vi "Limit Record Length.vi"(0 "Scope Reference":refnum<k15>, 11 "error in (no error)":errorcluster) -> (4 "Scope Reference Out":refnum<k15>, 15 "error out":errorcluster)   [LabVIEW 2020, in "LDO PSRR.lvlib"]
uses:
  LDO PSRR.lvlib
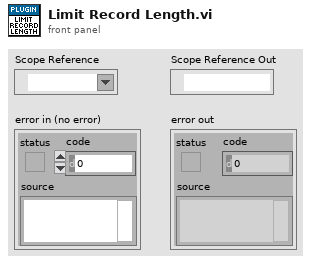
[diagram p1: front panel]
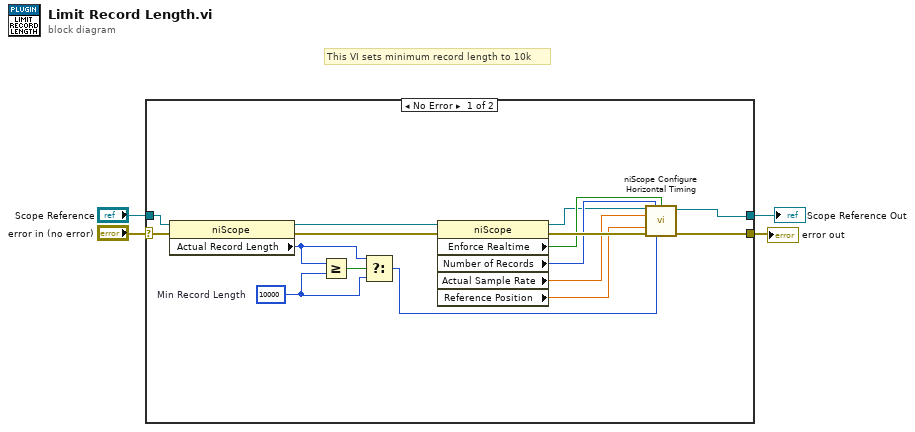
[diagram p0: block diagram]
diagram:
  # "This VI sets minimum record length to 10k"
  n1 = case shown="No Error" "error in (no error)" {
    selector: "error in (no error)" -> [w20 w22]
    tunnel: [w8 w22] -> w4
    tunnel: [w10 w21] -> w2
    tunnel: "Scope Reference" -> [w19 w21]
    frame No Error {
      w17 = 10000  # Min Record Length
      n2 = property class="niScope"(reference=w19, error in=w20) -> (reference out=w11:refnum<k15>, error out=w9:errorcluster, "Actual Record Length"=w6:i32)
      n3 = Greater Or Equal?(x=w6, y=w17) -> (x >= y?=w18:bool)
      n4 = Select(t=w6, s=w18, f=w17) -> (s? t:f=w7:i32)
      n5 = property class="niScope"(reference=w11, error in=w9) -> (reference out=w12:refnum<k15>, error out=w16:errorcluster, "Enforce Realtime"=w15:bool, "Number of Records"=w14:i32, "Actual Sample Rate"=w5:dbl, "Reference Position"=w13:dbl)
      n6 = call <instrlib>:"niScope Configure Horizontal Timing.vi"("instrument handle"=w12, "number of records"=w14, "enforce realtime"=w15, "min sample rate"=w5, "reference position"=w13, "error in"=w16, "min record length"=w7) -> ("instrument handle out"=w10:refnum<k15>, "error out"=w8:errorcluster)  [unwired: 7 in]
    }
    frame Error {
    }
  }
  "error out" <- w4
  "Scope Reference Out" <- w2
